vi "ABB Test report .vi"() -> (0 "error out":errorcluster)   [LabVIEW 2017]
uses:
  ABB global.vi
  <vilib>/Utility/NIReport.llb/NI_report.lvclass
panel:
  out "result string":string
  in  "Save":bool
  in  "View Pages":bool
  in  "Select page":u16(ring) items=["Cover Page", "Contents", "Pass/Fail Criteria", "Rated Data", " General Information", "Measurements", "No Load Test", "Short Circuit Test", "Heat Run", "Heat Run Data", "Cooling curve", "No Load Heat Run", "Heat Run Data", "No Load Cooling curve", "Bearing Run", "Bearing Run Data", "Efficiency", "Noise", "Noise Analysis 1", "Noise Analysis 2", "Bearing Inspection", "Instruments"]
  out "Message":string="Compiling Report...."
  in  "Select None":bool
  in  "Select All":bool
  out "Pages":string[](array[string])
  in  "Include":bool[](array[boolean])
  in  "Exit":bool
  in  "Print":bool
  in  "WebBrowser":refnum<k7>(container)
  # "Test Report"
  # "Include pages"
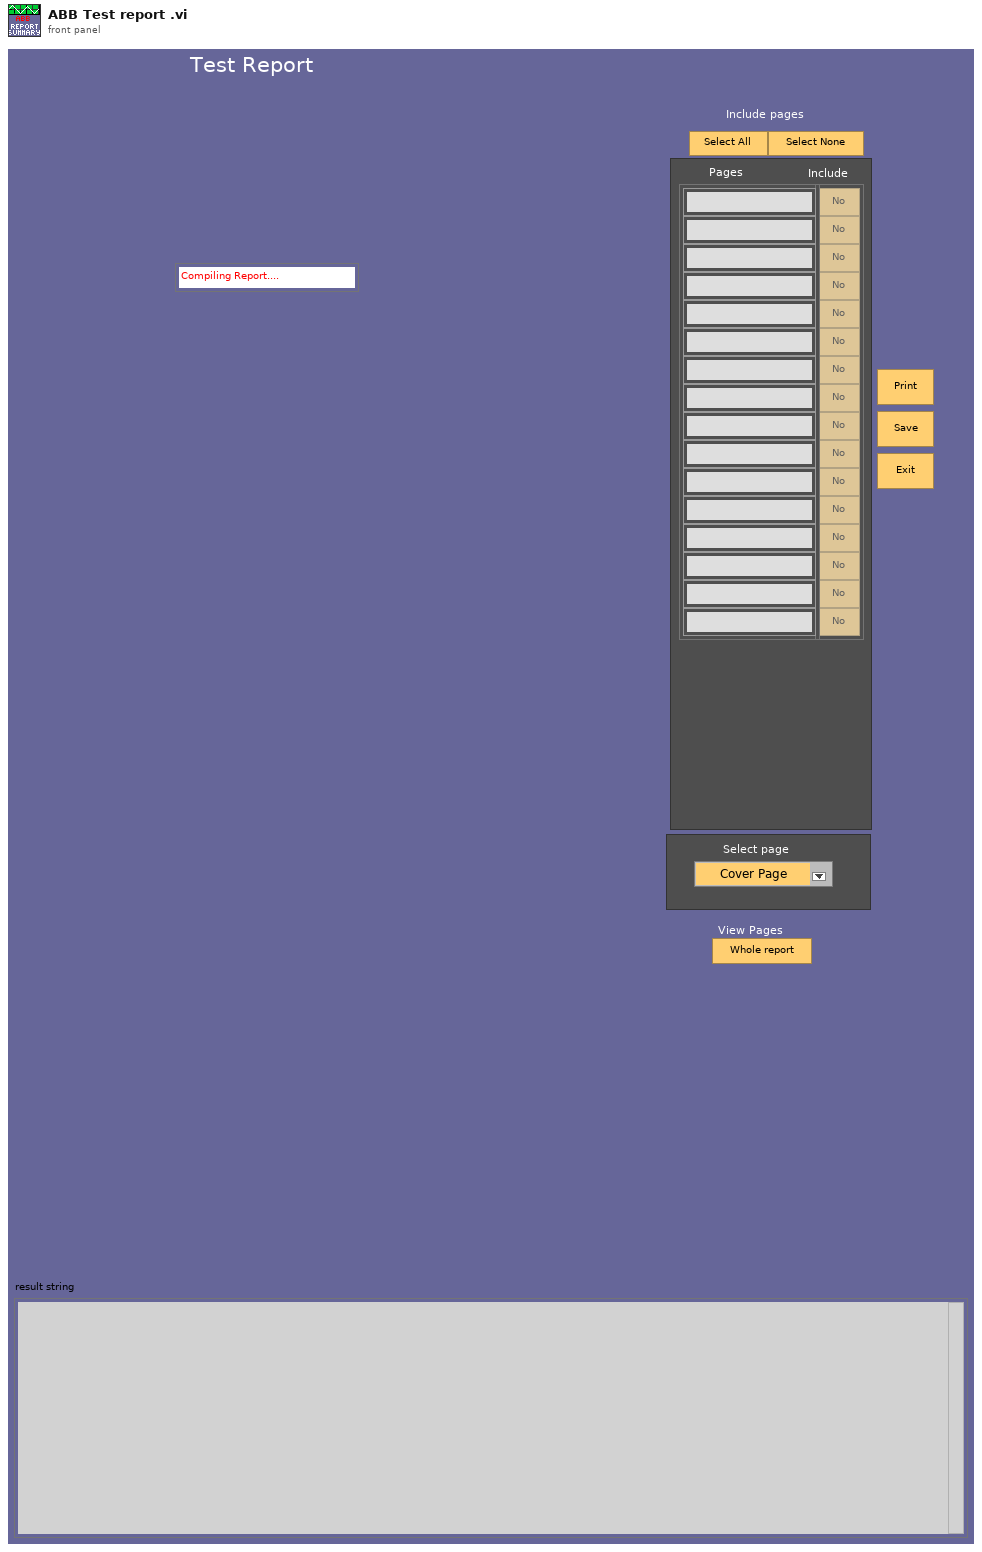
[diagram p1: front panel]
types:
  T1 = typedef "Generate Report Object Reference.ctl" = refnum<class "NI_report.lvclass">
  T2 = enum32{"existing file", "new file", "new or existing file", "existing dir", "new dir", "new or existing dir", "existing file (use LLBs)", "new file (use LLBs)", "new or existing file (use LLBs)", "new or existing file or directory (use LLBs)"}
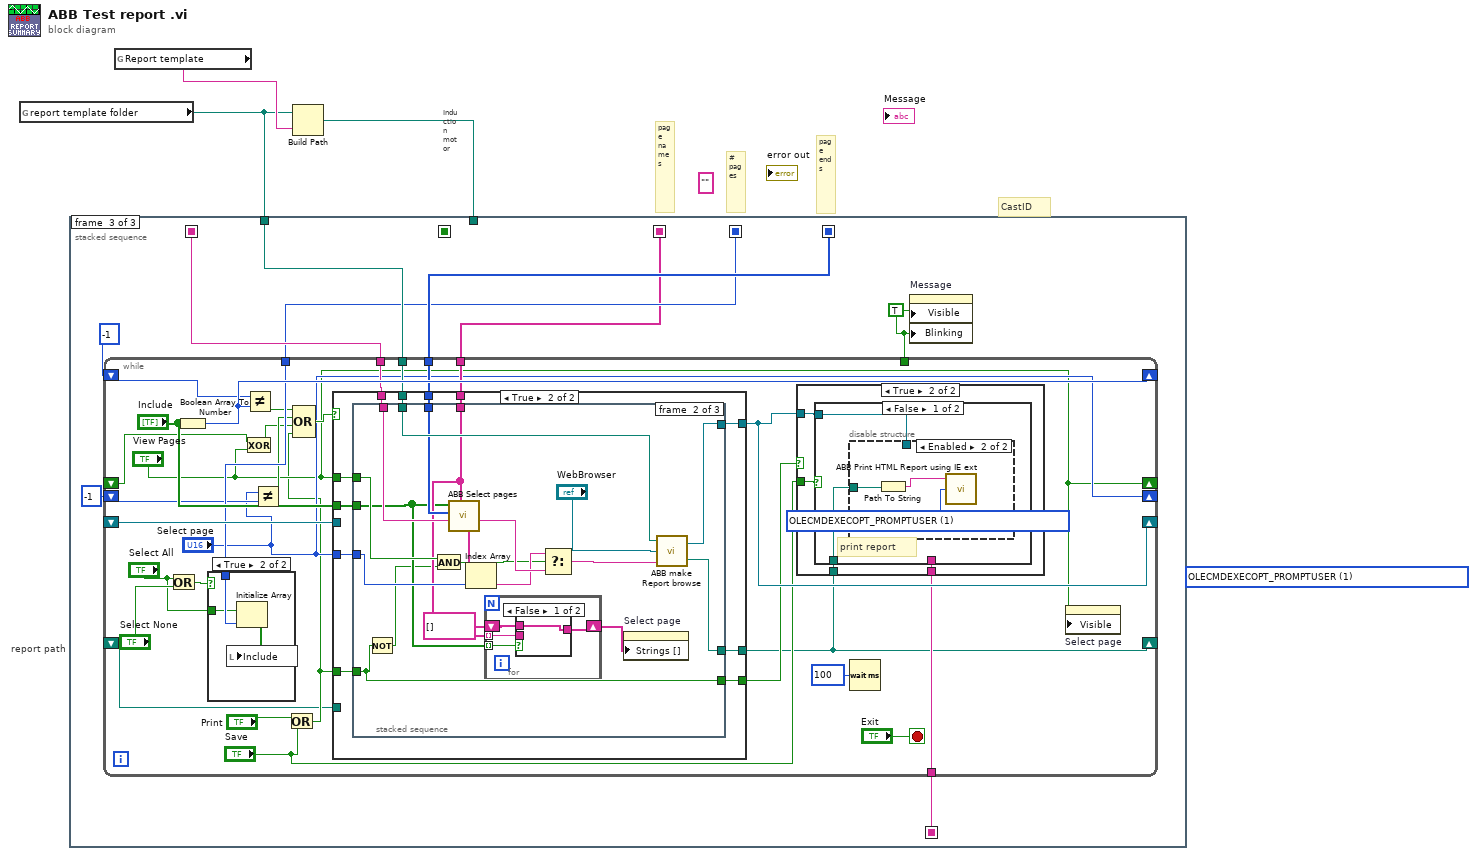
[diagram p0: block diagram]
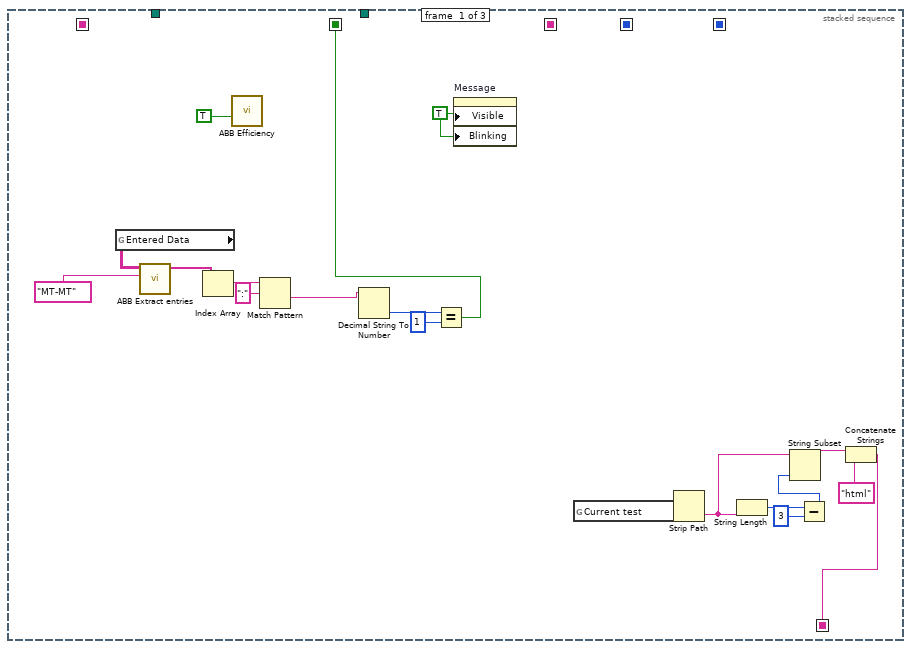
[diagram p2: hidden frame]
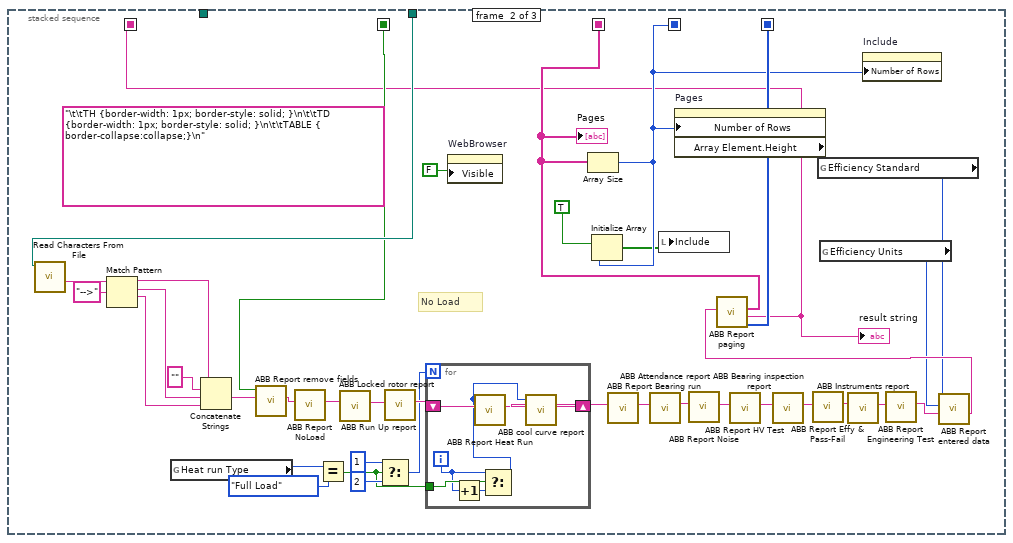
[diagram p3: hidden frame]
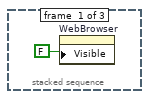
[diagram p6: hidden frame]
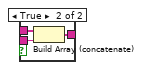
[diagram p7: hidden frame]
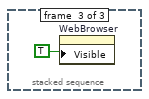
[diagram p8: hidden frame]
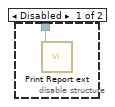
[diagram p10: hidden frame]
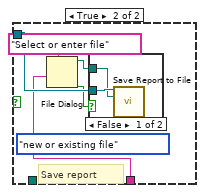
[diagram p11: hidden frame]
diagram:
  (unwired) 1 items=["OLECMDEXECOPT_DODEFAULT", "OLECMDEXECOPT_PROMPTUSER", "OLECMDEXECOPT_DONTPROMPTUSER", "OLECMDEXECOPT_SHOWHELP"] ("IE Print Options")
  (unwired) "" ("result string")
  # "report path"
  # "Induction motor"
  # "page names"
  # "# pages"
  # "page ends"
  # "CastID"
  n1 = global read "ABB global.vi" "report template folder"() -> (w1:path)
  n2 = global read "ABB global.vi" "Report template"() -> (w2:string)
  n3 = Build Path(base path=w1, name or relative path=w2) -> (appended path=w3:path)
  n4 = stacked-sequence {
    seq-local: [_ w30 _] -> [_ _ w75]
    seq-local: [_ w52 _] -> [_ _ w73]
    seq-local: [_ w51 _] -> [_ _ w72]
    seq-local: [_ w47 _] -> [_ _ w71]
    seq-local: [w12 _ _] -> [_ w34 _]
    seq-local: [w4 _ _] -> [_ _ w68]
    tunnel: w3 -> [_ w55 _]
    tunnel: w1 -> [_ _ w74]
    frame #0 {
      w22 = TRUE ("Visible")
      n5 = global read "ABB global.vi" "Entered Data"() -> (w20:string[][])
      n6 = call "ABB Extract entries.vi"("Entry ID"="MT-MT", "Entry table in"=w20) -> ("Selected Entries"=w18:string[])  [unwired: 9 in]
      n7 = Index Array(array=w18) -> (element=w17:string)  [unwired: 1 in]
      n8 = call "ABB Efficiency.vi"("auto save"=TRUE) -> ()  [unwired: 11 in]
      n9 = Match Pattern(string=w17, regular expression=":") -> (after substring=w15:string)  [unwired: 1 in, 3 out]
      n10 = Decimal String To Number(string=w15) -> (number=w14:i32)  [unwired: 2 in, 1 out]
      n11 = Equal?(x=w14, y=1) -> (x = y?=w12:bool)
      n12 = property on="Message" class="Str"("Visible"=w22, "Blinking"=w22) -> ()  [unwired: 2 in, 2 out]
      n13 = global read "ABB global.vi" "Current test"() -> (w11:path)
      n14 = Strip Path(path=w11) -> (name=w8:string)  [unwired: 1 out]
      n15 = String Length(string=w8) -> (length=w10:i32)
      n16 = Subtract(x=w10, y=3) -> (x-y=w7:i32)
      n17 = String Subset(string=w8, length (rest)=w7) -> (substring=w6:string)  [unwired: 1 in]
      n18 = Concatenate Strings(w6, "html" ("string")) -> (w4:string)
    }
    frame #1 {
      (unwired) "\t\tTH {border-width: 1px; border-style: solid; }\n\t\tTD {border-width: 1px; border-style: solid; }\n\t\tTABLE { border-collapse:collapse;}\n"
      # "No Load"
      n19 = call <vilib>:"Read Characters From File.vi"("file path (dialog if empty)"=w55) -> ("character string"=w60:string)  [unwired: 5 in, 3 out]
      n20 = Match Pattern(string=w60, regular expression="-->") -> (before substring=w58:string, match substring=w57:string, after substring=w56:string)  [unwired: 1 in, 1 out]
      n21 = global read "ABB global.vi" "Heat run Type"() -> (w42:enum16{"Full Load", "Partial- & No-Load"})
      n22 = Concatenate Strings(w58, "" ("string"), w57, w56) -> (w35:string)
      n23 = call "ABB Report remove fields.vi"("Report in"=w35, "Induction motor"=w34) -> ("Report out"=w26:string)  [unwired: 9 in]
      n24 = call "ABB Report NoLoad.vi"("Report in"=w26) -> ("Report out"=w45:string)  [unwired: 9 in, 1 out]
      n25 = Equal?(x=w42, y=enum16{"Full Load", "Partial Load"}."Full Load") -> (x = y?=w37:bool)
      n26 = call "ABB Locked rotor report.vi"("Report in"=w45) -> ("Report out"=w54:string)  [unwired: 9 in, 1 out]
      n27 = Select(t=1, s=w37, f=2) -> (s? t:f=w38:i32)
      n28 = call "ABB Run Up report.vi"("Report in"=w54) -> ("Report out"=w46:string)  [unwired: 10 in]
      n29 = for {
        N: w38 -> [_]
        shift-right: [w63] -> w27
        shift-left: w46 -> [w67]
        tunnel: w37 -> [w66]
        i -> [w65]
        n30 = Increment(x=w65) -> (x+1=w64:i32)
        n31 = Select(t=w65, s=w66, f=w64) -> (s? t:f=w61:i32)
        n32 = call "ABB Report Heat Run.vi"("Report in"=w67, "Heat run #"=w61) -> ("Report out"=w62:string)  [unwired: 9 in]
        n33 = call "ABB cool curve report.vi"("Report in"=w62, "Heat run #"=w61) -> ("Report out"=w63:string)  [unwired: 9 in]
      }
      n34 = property on="WebBrowser" class="AXCont"("Visible"=FALSE) -> ()  [unwired: 2 in, 2 out]
      n35 = call "ABB Report Bearing run.vi"("Report in"=w27) -> ("Report out"=w48:string)  [unwired: 10 in]
      n36 = call "ABB Attendance report.vi"("Report in"=w48) -> ("Report out"=w36:string)  [unwired: 10 in]
      n37 = call "ABB Report Noise.vi"("Report in"=w36) -> ("Report out"=w44:string)  [unwired: 10 in]
      n38 = call "ABB Report HV Test.vi"("Report in"=w44) -> ("Report out"=w32:string)  [unwired: 10 in]
      n39 = call "ABB Bearing inspection report.vi"("Report in"=w32) -> ("Report out"=w25:string)  [unwired: 10 in]
      n40 = call "ABB Report Effy & Pass-Fail.vi"("Report in"=w25) -> ("Report out"=w31:string)  [unwired: 10 in]
      n41 = global read "ABB global.vi" "Efficiency Standard"() -> (w24:u16)
      n42 = global read "ABB global.vi" "Efficiency Units"() -> (w23:u16)
      n43 = call "ABB Instruments report.vi"("Report in"=w31) -> ("Report out"=w29:string)  [unwired: 10 in]
      n44 = call "ABB Report Engineering Test.vi"("Report in"=w29) -> ("Report out"=w28:string)  [unwired: 10 in]
      n45 = call "ABB Report entered data.vi"("result string in"=w28, "Efficiency Units"=w23, "Efficiency Standard"=w24) -> ("result string out"=w33:string)  [unwired: 8 in]
      n46 = call "ABB Report paging.vi"("String"=w33) -> ("page ends"=w52:i32[], "result string"=w30:string, "Page Names"=w47:string[])  [unwired: 7 in, 1 out]
      "result string" <- w30
      "Pages" <- w47
      n47 = Array Size(array=w47) -> (size(s)=w51:i32)
      n48 = Initialize Array(TRUE, w51) -> (w50:bool[])
      n49 = local write "Include"(w50) -> ()
      n50 = property on="Pages" class="Arr (strict)" props=["Number of Rows", "Array Element", "Height"]("Number of Rows"=w51) -> ()  [unwired: 2 in, 3 out]
      n51 = property on="Include" class="Arr (strict)"("Number of Rows"=w51) -> ()  [unwired: 2 in, 2 out]
    }
    frame #2 {
      w70 = TRUE ("Visible")
      n52 = while {
        shift-right: [w105] -> _
        shift-left: -1 -> [w104]
        tunnel: w75 -> [w102]
        tunnel: w74 -> [w103]
        shift-right: [w101] -> _
        shift-left: _ -> [w100]
        tunnel: w73 -> [w98]
        tunnel: w72 -> [w95]
        tunnel: w71 -> [w92]
        tunnel: w70 -> [_]
        shift-right: ["Select page"] -> _
        shift-left: -1 ("index") -> [w89]
        shift-right: ["View Pages"] -> _
        shift-left: _ -> [w86]
        tunnel: w68 -> [w79]
        shift-right: [w77] -> _
        shift-left: _ -> [w78]
        stop <- "Exit" stop-if-true
        n53 = Or(x="Select All", y="Select None") -> (x .or. y?=w93:bool)
        n54 = Boolean Array To Number(Boolean array="Include") -> (number=w105:u32)
        n55 = case shown="True" w93 {
          tunnel: w95 -> [_ w109]
          tunnel: "Select All" -> [_ w108]
          frame False {
          }
          frame True {
            n56 = Initialize Array(w108, w109) -> (w107:bool[])
            n57 = local write "Include"(w107) -> ()
          }
        }
        n58 = Exclusive Or(1:"View Pages", 2:w86) -> (0:w85:bool)
        n59 = Not Equal?(x=w104, y=w105) -> (x != y?=w90:bool)
        n60 = Not Equal?(x="Select page", y=w89) -> (x != y?=w88:bool)
        n61 = Or(x="Print", y="Save") -> (x .or. y?=w82:bool)
        n62 = Compound Arithmetic op=OR(w90, w88, w85, w82) -> (w91:bool)
        n63 = case shown="True" w91 {
          tunnel: w103 -> [_ w123]
          tunnel: w102 -> [_ w121]
          tunnel: [w112 w122] -> w101
          tunnel: w100 -> [w112 _]
          tunnel: "Include" -> [_ w120]
          tunnel: w98 -> [_ w119]
          tunnel: w92 -> [_ w118]
          tunnel: "View Pages" -> [_ w117]
          tunnel: "Select page" -> [_ w116]
          tunnel: w82 -> [w111 w115]
          tunnel: [w111 w114] -> w83
          tunnel: [w110 w113] -> w77
          tunnel: w78 -> [w110 _]
          frame False {
          }
          frame True {
            n64 = stacked-sequence {
              tunnel: w123 -> [_ w142 _]
              tunnel: [_ w141 _] -> w122
              tunnel: w121 -> [_ w140 _]
              tunnel: w120 -> [_ w131 _]
              tunnel: w119 -> [_ w139 _]
              tunnel: w118 -> [_ w132 _]
              tunnel: w117 -> [_ w134 _]
              tunnel: w116 -> [_ w133 _]
              tunnel: w115 -> [_ w126 _]
              tunnel: [_ w126 _] -> w114
              tunnel: [_ w125 _] -> w113
              frame #0 {
                n65 = property on="WebBrowser" class="AXCont"("Visible"=FALSE) -> ()  [unwired: 2 in, 2 out]
              }
              frame #1 {
                n66 = Not(x=w126) -> (.not. x?=w127:bool)
                n67 = And(x=w134, y=w127) -> (x .and. y?=w128:bool)
                n68 = call "ABB Select pages.vi"("Page Names"=w132, "Report in"=w140, "Page ends"=w139, "Page select"=w131) -> ("Report out"=w138:string, "Pages out"=w136:string[])  [unwired: 5 in, 1 out]
                n69 = Index Array(array=w136, index=w133) -> (element=w135:string)
                n70 = for {
                  tunnel: w132 -> [w146] mode=indexing
                  tunnel: w131 -> [w147] mode=indexing
                  shift-right: [w144] -> w129
                  shift-left: string[] [] -> [w145]
                  n71 = case shown="False" w147 {
                    tunnel: w146 -> [_ w151]
                    tunnel: w145 -> [w148 w150]
                    tunnel: [w148 w149] -> w144
                    frame False {
                    }
                    frame True {
                      n72 = Build Array (concatenate)(w150, w151) -> (w149:string[])
                    }
                  }
                }
                n73 = Select(t=w135, s=w128, f=w138) -> (s? t:f=w137:string)
                n74 = property on="Select page" class="Ring (strict)"("Strings []"=w129) -> ()  [unwired: 2 in, 2 out]
                n75 = call "ABB make Report browse.vi"("result string"=w137, "WebBrowser"="WebBrowser", "report template folder"=w142) -> ("Report  path"=w125:path, "report out"=w141:T1)
              }
              frame #2 {
                n76 = property on="WebBrowser" class="AXCont"("Visible"=TRUE) -> ()  [unwired: 2 in, 2 out]
              }
            }
          }
        }
        n77 = case shown="True" w83 {
          tunnel: w101 -> [_ w156]
          tunnel: "Save" -> [_ w155]
          tunnel: w79 -> [_ w154]
          tunnel: w77 -> [_ w153]
          frame False {
          }
          frame True {
            n78 = case shown="False" w155 {
              tunnel: w156 -> [w158 w167]
              tunnel: w154 -> [_ w166]
              tunnel: w153 -> [w157 _]
              frame False {
                # "print report"
                n79 = disable-structure shown="Enabled" {
                  disable-tunnel: w158 -> [w159 _]
                  disable-tunnel: w157 -> [_ w162]
                  frame Disabled {
                    n80 = call "Print Report ext.vi"("report in"=w159) -> ()  [unwired: 6 in, 2 out]
                  }
                  frame Enabled {
                    w160 = 1 items=["OLECMDEXECOPT_DODEFAULT", "OLECMDEXECOPT_PROMPTUSER", "OLECMDEXECOPT_DONTPROMPTUSER", "OLECMDEXECOPT_SHOWHELP"] ("IE Print Options")
                    n81 = Path To String(path=w162) -> (string=w161:string)
                    n82 = call "ABB Print HTML Report using IE ext.vi"("IE Print Options"=w160, "Path to HTML"=w161) -> ()  [unwired: 3 in, 1 out]
                  }
                }
              }
              frame True {
                (unwired) T2."new or existing file" ("select mode (2)")
                # "Save report"
                n83 = File Dialog(7:"Select or enter file" ("prompt"), 9:w166) -> (1:w163:bool, 3:w164:path)  [unwired: 5 in, 2 out]
                n84 = case shown="False" w163 {
                  tunnel: w167 -> [w169 _]
                  tunnel: w164 -> [w168 _]
                  frame False {
                    n85 = call-dynamic "Save Report to File.vi"("report in"=w169, "report file path"=w168) -> ()  [unwired: 12 in, 2 out]
                  }
                  frame True {
                  }
                }
              }
            }
          }
        }
        n86 = Wait (ms)(milliseconds to wait=u32 100) -> ()  [unwired: 1 out]
        n87 = property on="Select page" class="Ring (strict)"("Visible"="View Pages") -> ()  [unwired: 2 in, 2 out]
      }
      n88 = property on="Message" class="Str"("Visible"=w70, "Blinking"=w70) -> ()  [unwired: 2 in, 2 out]
    }
  }
